vi "探测器列表-设备改名+移数据.vi"(5 "元素名[]-探测器信息":string[](array[string]), 7 "table名-探测器列表":string, 8 "error in (no error)":errorcluster, 10 "改名":cluster{"原名":string, "新名":string}, 11 "数据库引用":T1) -> (0 "error out":errorcluster, 3 "数据库连接引用out":T1)   [LabVIEW 2017]
uses:
  <vilib>/addons/database/Connection.llb/Conn ObjectReference.ctl
  <vilib>/addons/database/NI_Database_API.lvlib
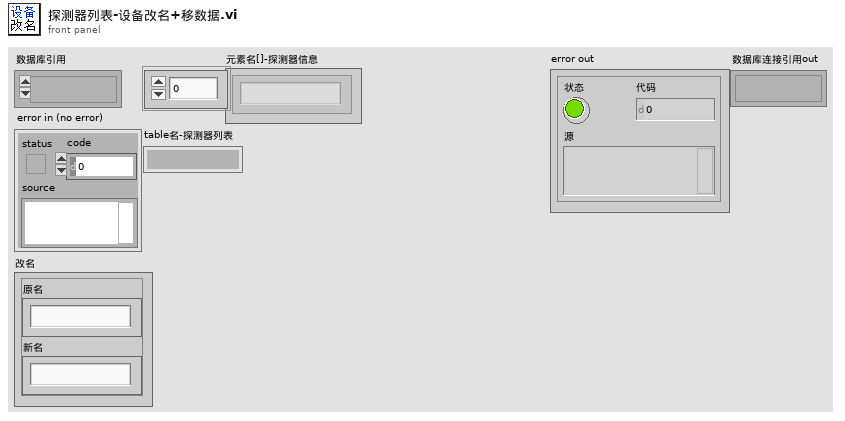
[diagram p1: front panel]
types:
  T1 = typedef "NI_Database_API.lvlib/Conn ObjectReference.ctl" = refnum<k1>
  T2 = typedef "探测器信息.ctl" = cluster{"网络地址":string, "名称":string, "备注":string, "累积剂量":dbl, "累积限值":dbl, "硬件剂量率限值":T3, "剂量率限值1":dbl, "剂量率限值2":dbl, "报警方式":T4}
  T3 = typedef "探头剂量率限值选择.ctl" = enum16{"一级限值", "二级限值"}
  T4 = typedef "报警方式选择.ctl" = enum16{"常报警", "自动静音", "手动静音"}
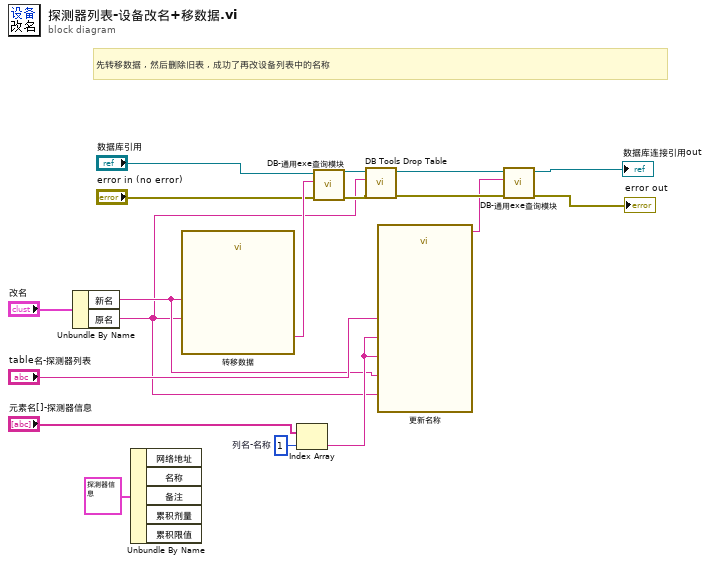
[diagram p0: block diagram]
diagram:
  w9 = 1  # 列名-名称
  # "先转移数据 , 然后删除旧表 , 成功了再改设备列表中的名称"
  n1 = Unbundle By Name("改名") -> ("新名"=w4:string, "原名"=w3:string)
  n2 = Unbundle By Name(T2 {"网络地址"="", "名称"="", "备注"="", "累积剂量"=0.0, "累积限值"=0.0, "硬件剂量率限值"=enum."一级限值", "剂量率限值1"=0.0, "剂量率限值2"=0.0, "报警方式"=enum."常报警"} ("输入簇")) -> ()  [unwired: 5 out]
  n3 = call "转移数据"("表名-新数据表名称"=w4, "表名-原数据表名称"=w3) -> ("Result"=w18:string)  [unwired: 12 in, 1 out]
  n4 = Index Array(array="元素名[]-探测器信息", index=w9) -> (element=w7:string)
  n5 = call "DB-通用exe查询模块.vi"("error in (no error)"="error in (no error)", "SQL query"=w18, "数据库连接引用"="数据库引用") -> ("error out"=w15:errorcluster, "数据库连接引用out"=w16:T1)  [unwired: 4 in, 3 out]
  n6 = call <vilib>:"DB Tools Drop Table.vi"("error in (no error)"=w15, "table"=w3, "connection reference"=w16) -> ("error out"=w13:errorcluster, "connection reference out"=w12:T1)  [unwired: 5 in]
  n7 = call "更新名称"("列名-名称1"=w7, "表名-设备表"="table名-探测器列表", "列名-名称"=w7, "新设备名称"=w4, "原设备名称"=w3) -> ("Result"=w11:string)  [unwired: 9 in, 1 out]
  n8 = call "DB-通用exe查询模块.vi"("error in (no error)"=w13, "SQL query"=w11, "数据库连接引用"=w12) -> ("error out"=→"error out":errorcluster, "数据库连接引用out"=→"数据库连接引用out":T1)  [unwired: 4 in, 3 out]
